vi "MGCC_MdlMgmt_MovetonewMicrogrid.vi"() -> (0 "error out":errorcluster, 1 "error out 2":errorcluster)   [LabVIEW 2016]
uses:
  Global_MdlMgmt.vi
  <vilib>/imath/engines/lvmath2/RunTimeEngine/IndexRead/NIMS M($,R2).vi
  <instcachedir>/0/NIMS M($,R2)_D9380E19261A4ADFB2D364AF6959C6EF.lvgen/NIMS M($,R2)_D9380E19261A4ADFB2D364AF6959C6EF_001.vi
  <vilib>/imath/engines/lvmath2/RunTimeEngine/BuiltInFunctions/max/1 input/NIMS_max(RM).vi
  <instcachedir>/0/NIMS_max(RM)_358AE92FF7FA4D91BF0D9DEC69043403.lvgen/NIMS_max(RM)_358AE92FF7FA4D91BF0D9DEC69043403_000.vi
  <vilib>/imath/engines/lvmath2/RunTimeEngine/BuiltInFunctions/max/1 input/NIMS_max(RV).vi
  <instcachedir>/0/NIMS_max(RV)_237633DB1D604D5BA7001287DF3C7957.lvgen/NIMS_max(RV)_237633DB1D604D5BA7001287DF3C7957_000.vi
  <vilib>/imathl/engines/lvmath/Functions/Error Handling/Create Error.vi
  <vilib>/imath/engines/lvmath2/RunTimeEngine/IndexRead/NIMS M($,S).vi
  <instcachedir>/0/NIMS M($,S)_3E5749BBB62E49528D4765A77F1F6D98.lvgen/NIMS M($,S)_3E5749BBB62E49528D4765A77F1F6D98_000.vi
  <vilib>/imath/engines/lvmath2/RunTimeEngine/BuiltInFunctions/length/NIMS_length(GV).vi
  <instcachedir>/0/NIMS_length(GV)_08A3D13377FD4E4B96F5795FBF3698FA.lvgen/NIMS_length(GV)_08A3D13377FD4E4B96F5795FBF3698FA_000.vi
  <instcachedir>/0/NIMS_length(GV)_08A3D13377FD4E4B96F5795FBF3698FA.lvgen/NIMS_length(GV)_08A3D13377FD4E4B96F5795FBF3698FA_002.vi
  <vilib>/imath/engines/lvmath2/RunTimeEngine/BuiltInFunctions/zeros/NIMS_M=zeros(I32,I32).vi
  <vilib>/imath/engines/lvmath2/RunTimeEngine/ErrorHandling/NIMS_Create Error From Enums.vi
  <vilib>/imath/engines/lvmath2/RunTimeEngine/IndexReplace/NIMS M(S,$)=V.vi
  <instcachedir>/0/NIMS M(S,$)=V_BCCFA522A894489B8FA760383D74A164.lvgen/NIMS M(S,$)=V_BCCFA522A894489B8FA760383D74A164_002.vi
  <vilib>/imath/engines/lvmath2/RunTimeEngine/BuiltInFunctions/zeros/NIMS_V=zeros(I32,I32).vi
  <vilib>/imath/engines/lvmath2/RunTimeEngine/RangeToken/NIMS_Range_R3 - Integer.vi
  <instcachedir>/0/NIMS_Range_R3 - Integer_A435E2FF893B4C718FD5055FE39FE2F6.lvgen/NIMS_Range_R3 - Integer_A435E2FF893B4C718FD5055FE39FE2F6_000.vi
  <vilib>/imath/engines/lvmath2/RunTimeEngine/CommandStatement/MC_CommandStatement_break.vi
  <vilib>/imath/engines/lvmath2/RunTimeEngine/IndexRead/NIMS M(S,R2).vi
  <instcachedir>/0/NIMS M(S,R2)_45730E4D0DB74D118F715F4F99DCE4D7.lvgen/NIMS M(S,R2)_45730E4D0DB74D118F715F4F99DCE4D7_000.vi
  <vilib>/imath/engines/lvmath2/RunTimeEngine/BuiltInFunctions/is_membermx/NIMS_is_membermx(GM,GM).vi
  <instcachedir>/0/NIMS_is_membermx(GM,GM)_DE25F6F493CE4EA1946032CBAF7A49B3.lvgen/NIMS_is_membermx(GM,GM)_DE25F6F493CE4EA1946032CBAF7A49B3_000.vi
  <vilib>/imath/engines/lvmath2/RunTimeEngine/BuiltInFunctions/sum/NIMS_sum(GM,Sca).vi
  <instcachedir>/0/NIMS_sum(GM,Sca)_79BF37D5D11844228B167097B6AFCFEB.lvgen/NIMS_sum(GM,Sca)_79BF37D5D11844228B167097B6AFCFEB_001.vi
  <vilib>/imath/engines/lvmath2/RunTimeEngine/IndexRead/NIMS M(S,S).vi
  <instcachedir>/0/NIMS M(S,S)_AC51E74150A542F7991B9634C66F3096.lvgen/NIMS M(S,S)_AC51E74150A542F7991B9634C66F3096_000.vi
  <vilib>/imath/engines/lvmath2/RunTimeEngine/IndexReplace/NIMS M(S,S)=S.vi
  <instcachedir>/0/NIMS M(S,S)=S_98E40400474E4398B113AE20298B4F82.lvgen/NIMS M(S,S)=S_98E40400474E4398B113AE20298B4F82_000.vi
  <vilib>/imath/engines/lvmath2/RunTimeEngine/BuiltInFunctions/sum/NIMS_sum(GV).vi
  <instcachedir>/0/NIMS_sum(GV)_67F5EC36BC034E54A6BEC5B0673C00E5.lvgen/NIMS_sum(GV)_67F5EC36BC034E54A6BEC5B0673C00E5_000.vi
  <vilib>/imath/engines/lvmath2/RunTimeEngine/BuiltInFunctions/findnz/NIMS_[1o]_findnz(GRowV).vi
  <instcachedir>/0/NIMS_[1o]_findnz(GRowV)_1AF74843B4874134ADE908C0A4A72F3C.lvgen/NIMS_[1o]_findnz(GRowV)_1AF74843B4874134ADE908C0A4A72F3C_000.vi
  <vilib>/imath/engines/lvmath2/RunTimeEngine/IndexRead/NIMS M($,V).vi
  <instcachedir>/0/NIMS M($,V)_706F2CE2C8E141269FD4C8A402E169C5.lvgen/NIMS M($,V)_706F2CE2C8E141269FD4C8A402E169C5_005.vi
  <vilib>/imath/engines/lvmath2/RunTimeSupport/NIMS_Get Any Vector_w Error - Matrix.vi
  <instcachedir>/0/NIMS_Get Any Vector_w Error - Matrix_2B7BCBEFD1FA4E1C95EFF9244314B21B.lvgen/NIMS_Get Any Vector_w Error - Matrix_2B7BCBEFD1FA4E1C95EFF9244314B21B_001.vi
  <vilib>/imath/engines/lvmath2/RunTimeEngine/BuiltInFunctions/sets_union/NIMS_sets_union(GV2).vi
  <instcachedir>/0/NIMS_sets_union(GV2)_D04DE11E528744D2B40881BC08732835.lvgen/NIMS_sets_union(GV2)_D04DE11E528744D2B40881BC08732835_007.vi
  <vilib>/imath/engines/lvmath2/RunTimeEngine/IndexReplace/NIMS M($,V)=V.vi
  <instcachedir>/0/NIMS M($,V)=V_456DED019FC24BEA8A1C4EECB3220DB5.lvgen/NIMS M($,V)=V_456DED019FC24BEA8A1C4EECB3220DB5_000.vi
  <vilib>/imath/engines/lvmath2/RunTimeEngine/RangeToken/NIMS_Range.vi
  <instcachedir>/0/NIMS_Range_A7C094595B484CA7AF10685B02D808ED.lvgen/NIMS_Range_A7C094595B484CA7AF10685B02D808ED_001.vi
  <vilib>/imath/engines/lvmath2/RunTimeEngine/NodeEndStatement/NIMS_NodeEndStatement_Output.vi
  <instcachedir>/0/NIMS_NodeEndStatement_Output_53EC0D466D134D7ABD903AC30B43404B.lvgen/NIMS_NodeEndStatement_Output_53EC0D466D134D7ABD903AC30B43404B_002.vi
  <instcachedir>/0/NIMS_NodeEndStatement_Output_53EC0D466D134D7ABD903AC30B43404B.lvgen/NIMS_NodeEndStatement_Output_53EC0D466D134D7ABD903AC30B43404B_011.vi
  <vilib>/imath/engines/lvmath2/RunTimeEngine/ErrorHandling/NIMS_Finalize Error.vi
  <vilib>/Utility/error.llb/Error Cluster From Error Code.vi
  <vilib>/ErrorRing/Error Ring.xnode
panel:
  out "subarray":cdb[](array[numeric])
  out "Nodematrix":dbl[][](array[numeric])
  out "island_number":i32
  out "Microgrid Topology Overall":dbl[][](array[numeric])
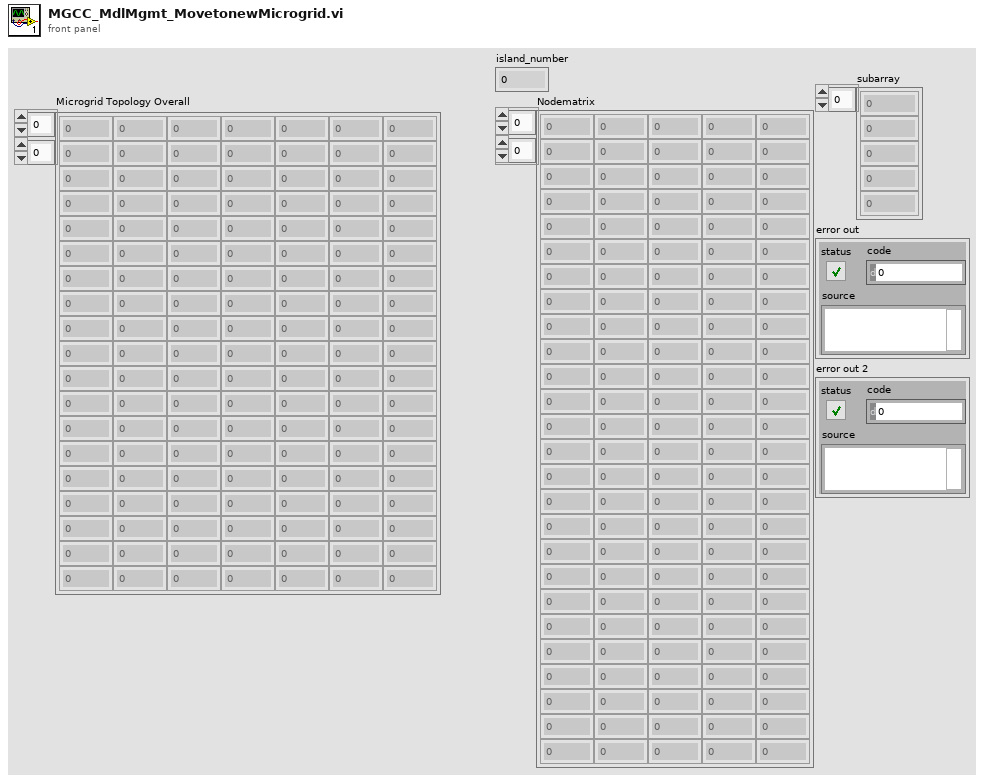
[diagram p1: front panel]
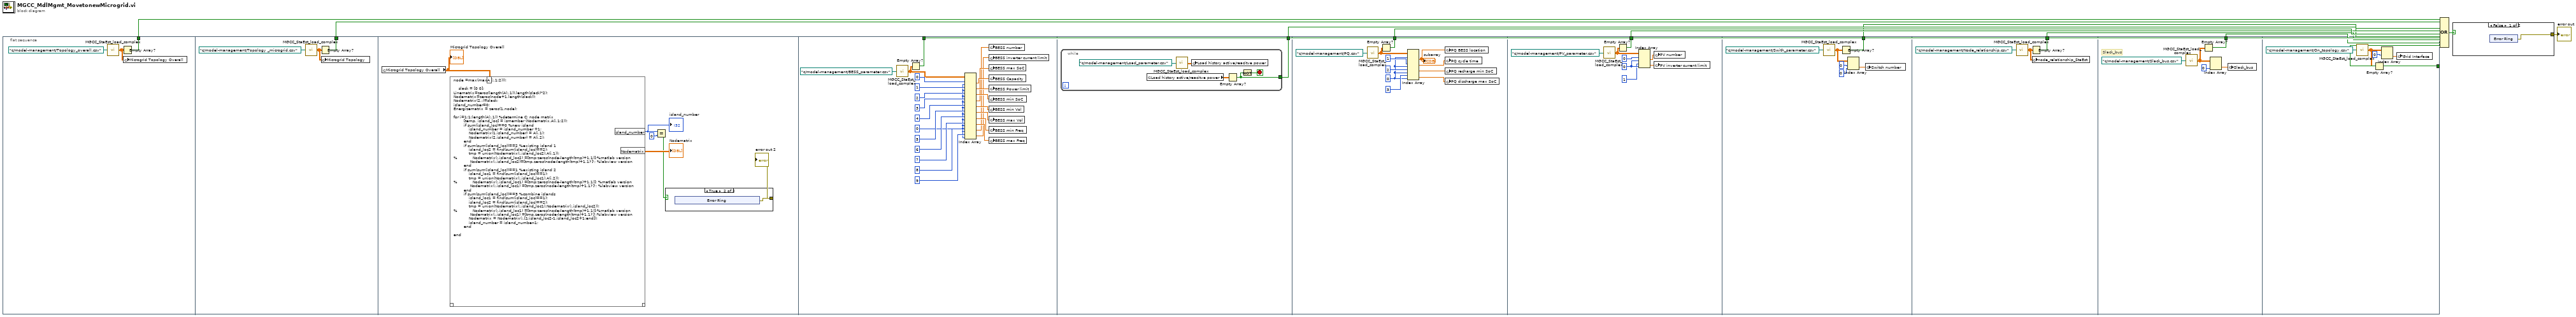
[diagram p0: block diagram]
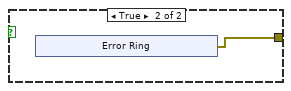
[diagram p2: hidden frame]
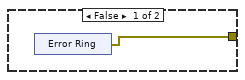
[diagram p3: hidden frame]
diagram:
  n1 = flat-sequence {
    tunnel: [w13] -> w12
    tunnel: [w16] -> w11
    tunnel: [w756] -> w10
    tunnel: [w780] -> w9
    tunnel: [w786] -> w7
    tunnel: [w797] -> w6
    tunnel: [w805] -> w5
    tunnel: [w811] -> w4
    tunnel: [w814] -> w3
    tunnel: [w819] -> w2
    frame #0 {
      n2 = call "MGCC_StaEst_load_complex.vi"("file path (dialog if empty)"=path "c:/model-management/Topology_overall.csv" ("file path (use dialog)")) -> ("Array 13"=w14:cdb[][])
      n3 = Empty Array?(array=w14) -> (empty?=w13:bool)
      n4 = global write "Global_MdlMgmt.vi" "Microgrid Topology Overall"(w14) -> ()
    }
    frame #1 {
      n5 = call "MGCC_StaEst_load_complex.vi"("file path (dialog if empty)"=path "c:/model-management/Topology _microgrid.csv" ("file path (use dialog)")) -> ("Array 13"=w17:cdb[][])
      n6 = Empty Array?(array=w17) -> (empty?=w16:bool)
      n7 = global write "Global_MdlMgmt.vi" "Microgrid Topology"(w17) -> ()
    }
    frame #2 {
      n8 = global read "Global_MdlMgmt.vi" "Microgrid Topology Overall"() -> (w24:dbl[][])
      "Microgrid Topology Overall" <- w24
      n9 = mathscript code="node =max(max(A(:,1:2)));\n\n    slack = [0 0];\nLinematrix=zeros(length(A(:,1)),length(slack)*2);\nNodematrix=zeros(node+1,length(slack));\nNodematrix(2,:)=slack;\nisland_number=0;\nEnergizematrix = zeros(1,node);\n\nfor i=1:1:length(A(:,1)) %determine C: node matrix\n        [temp, island_loc] = ismember (Nodematrix,A(i,1:2));\n        if sum(island_loc)==0 %new island\n            island_number = island_number +1;\n            Nodematrix(1,island_number) = A(i,1);\n            Nodematrix(2,island_number) = A(i,2);\n        end\n        if sum(sum(island_loc))==2 %existing island 1\n            island_loc2 = find(sum(island_loc)==2);\n            tmp = union(Nodematrix(:,island_loc2),A(i,1));\n%            Nodematrix(:,island_loc2) =[tmp;zeros(node-length(tmp)+1,1)];%matlab version\n             Nodematrix(:,island_loc2)=[tmp,zeros(node-length(tmp)+1,1)']'; %labview version\n        end\n        if sum(sum(island_loc))==1 %existing island 2\n            island_loc1 = find(sum(island_loc)==1);\n            tmp = union(Nodematrix(:,island_loc1),A(i,2));\n%            Nodematrix(:,island_loc1) =[tmp;zeros(node-length(tmp)+1,1)]; %matlab version\n             Nodematrix(:,island_loc1) =[tmp,zeros(node-length(tmp)+1,1)']'; %labview version\n        end\n        if sum(sum(island_loc))==3 %combine islands\n            island_loc1 = find(sum(island_loc)==1);\n            island_loc2 = find(sum(island_loc)==2);\n            tmp = union(Nodematrix(:,island_loc1),Nodematrix(:,island_loc2));\n%            Nodematrix(:,island_loc1) =[tmp;zeros(node-length(tmp)+1,1)];%matlab version\n             Nodematrix(:,island_loc1) =[tmp,zeros(node-length(tmp)+1,1)']';%labview version\n            Nodematrix = Nodematrix(:,[1:island_loc2-1,island_loc2+1:end]);\n            island_number = island_number-1;\n        end\n\nend"("A"=w24) -> ("island_number"=w22:i32, "Nodematrix"=→"Nodematrix":dbl[][])  [unwired: 1 in, 1 out]
      "island_number" <- w22
      n10 = Equal?(x=w22, y=0) -> (x = y?=w20:bool)
      n11 = case shown="True" w20 {
        tunnel: [w25 w27] -> w19
        frame False {
          n12 = xnode "Error Ring"() -> ("error out"=w25:errorcluster)
        }
        frame True {
          n13 = xnode "Error Ring"() -> ("error out"=w27:errorcluster)
        }
      }
      "error out 2" <- w19
    }
    frame #3 {
      w768 = 0
      n14 = call "MGCC_StaEst_load_complex.vi"("file path (dialog if empty)"=path "c:/model-management/BESS_parameter.csv" ("file path (use dialog)")) -> ("Array 13"=w757:cdb[][])
      n15 = Empty Array?(array=w757) -> (empty?=w756:bool)
      n16 = Index Array(array=w757, index (row) #1=0 ("disabled index (row)"), index (col) #1=w768, index (row) #2=1 ("disabled index (row)"), index (col) #2=w768, index (row) #3=2 ("disabled index (row)"), index (col) #3=w768, index (row) #4=3 ("disabled index (row)"), index (col) #4=w768, index (row) #5=4 ("disabled index (row)"), index (col) #5=w768, index (row) #6=5 ("disabled index (row)"), index (col) #6=w768, index (row) #7=6 ("disabled index (row)"), index (col) #7=w768, index (row) #8=7 ("index (row)"), index (col) #8=w768, index (row) #9=8 ("index (row)"), index (col) #9=w768, index (row) #10=9 ("index (row)"), index (col) #10=w768) -> (element #1=w767:cdb, element #2=w766:cdb, element #3=w765:cdb, element #4=w764:cdb, element #5=w763:cdb, element #6=w762:cdb, element #7=w761:cdb, element #8=w760:cdb, element #9=w759:cdb, element #10=w758:cdb)
      n17 = global write "Global_MdlMgmt.vi" "BESS number"(w759) -> ()
      n18 = global write "Global_MdlMgmt.vi" "BESS inverter current limit"(w758) -> ()
      n19 = global write "Global_MdlMgmt.vi" "BESS max SoC"(w764) -> ()
      n20 = global write "Global_MdlMgmt.vi" "BESS Capacity"(w767) -> ()
      n21 = global write "Global_MdlMgmt.vi" "BESS Power limit"(w766) -> ()
      n22 = global write "Global_MdlMgmt.vi" "BESS min SoC"(w765) -> ()
      n23 = global write "Global_MdlMgmt.vi" "BESS min Vol"(w763) -> ()
      n24 = global write "Global_MdlMgmt.vi" "BESS max Vol"(w762) -> ()
      n25 = global write "Global_MdlMgmt.vi" "BESS min Freq"(w761) -> ()
      n26 = global write "Global_MdlMgmt.vi" "BESS max Freq"(w760) -> ()
    }
    frame #4 {
      n27 = while {
        tunnel: [w781] -> w780
        stop <- w782 stop-if-true
        n28 = global read "Global_MdlMgmt.vi" "Load history active/reacitve power"() -> (w783:dbl[][])
        n29 = call "MGCC_StaEst_load_complex.vi"("file path (dialog if empty)"=path "c:/model-management/Load_parameter.csv" ("file path (use dialog)")) -> ("Array 13"=w784:cdb[][])
        n30 = global write "Global_MdlMgmt.vi" "Load history active/reacitve power"(w784) -> ()
        n31 = Empty Array?(array=w783) -> (empty?=w781:bool)
        n32 = Not(x=w781) -> (.not. x?=w782:bool)
      }
    }
    frame #5 {
      w788 = 0
      n33 = call "MGCC_StaEst_load_complex.vi"("file path (dialog if empty)"=path "c:/model-management/PQ.csv" ("file path (use dialog)")) -> ("Array 13"=w787:cdb[][])
      n34 = Empty Array?(array=w787) -> (empty?=w786:bool)
      n35 = Index Array(array=w787, index (row) #1=w788, index (row) #2=1 ("disabled index (row)"), index (col) #2=w788, index (row) #3=2 ("disabled index (row)"), index (col) #3=w788, index (row) #4=3 ("disabled index (row)"), index (col) #4=w788) -> (element #1=w792:cdb[], element #2=w791:cdb, element #3=w790:cdb, element #4=w789:cdb)  [unwired: 1 in]
      "subarray" <- w792
      n36 = global write "Global_MdlMgmt.vi" "PQ BESS location"(w792) -> ()
      n37 = global write "Global_MdlMgmt.vi" "PQ cycle time"(w791) -> ()
      n38 = global write "Global_MdlMgmt.vi" "PQ recharge min SoC"(w790) -> ()
      n39 = global write "Global_MdlMgmt.vi" "PQ discharge max SoC"(w789) -> ()
    }
    frame #6 {
      w803 = 0
      n40 = call "MGCC_StaEst_load_complex.vi"("file path (dialog if empty)"=path "c:/model-management/PV_parameter.csv" ("file path (use dialog)")) -> ("Array 13"=w798:cdb[][])
      n41 = Empty Array?(array=w798) -> (empty?=w797:bool)
      n42 = Index Array(array=w798, index (row) #1=0 ("disabled index (row)"), index (col) #1=w803, index (row) #2=1 ("disabled index (row)"), index (col) #2=w803) -> (element #1=w800:cdb, element #2=w799:cdb)
      n43 = global write "Global_MdlMgmt.vi" "PV number"(w800) -> ()
      n44 = global write "Global_MdlMgmt.vi" "PV inverter current limit"(w799) -> ()
    }
    frame #7 {
      n45 = call "MGCC_StaEst_load_complex.vi"("file path (dialog if empty)"=path "c:/model-management/Swith_parameter.csv" ("file path (use dialog)")) -> ("Array 13"=w806:cdb[][])
      n46 = Empty Array?(array=w806) -> (empty?=w805:bool)
      n47 = Index Array(array=w806, index (row)=0, index (col)=0 ("disabled index (col)")) -> (element=w807:cdb)
      n48 = global write "Global_MdlMgmt.vi" "Switch number"(w807) -> ()
    }
    frame #8 {
      n49 = call "MGCC_StaEst_load_complex.vi"("file path (dialog if empty)"=path "c:/model-management/Node_relationship.csv" ("file path (use dialog)")) -> ("Array 13"=w812:cdb[][])
      n50 = Empty Array?(array=w812) -> (empty?=w811:bool)
      n51 = global write "Global_MdlMgmt.vi" "node_relationship_StaEst"(w812) -> ()
    }
    frame #9 {
      # "Slack_bus"
      n52 = call "MGCC_StaEst_load_complex.vi"("file path (dialog if empty)"=path "c:/model-management/Slack_bus.csv" ("file path (use dialog)")) -> ("Array 13"=w815:cdb[][])
      n53 = Empty Array?(array=w815) -> (empty?=w814:bool)
      n54 = Index Array(array=w815, index (col)=0 ("disabled index (col)")) -> (element=w816:cdb[])  [unwired: 1 in]
      n55 = global write "Global_MdlMgmt.vi" "Slack_bus"(w816) -> ()
    }
    frame #10 {
      n56 = call "MGCC_StaEst_load_complex.vi"("file path (dialog if empty)"=path "c:/model-management/On_topology.csv" ("file path (use dialog)")) -> ("Array 13"=w820:cdb[][])
      n57 = Empty Array?(array=w820) -> (empty?=w819:bool)
      n58 = Index Array(array=w820, index (row)=0) -> (element=w822:cdb[])  [unwired: 1 in]
      n59 = global write "Global_MdlMgmt.vi" "Grid Interface"(w822) -> ()
    }
  }
  n60 = Compound Arithmetic op=OR(w12, w11, w10, w9, w6, w7, w5, w4, w3, w2) -> (w8:bool)
  n61 = case shown="False" w8 {
    tunnel: [w824 w826] -> w1
    frame False {
      n62 = xnode "Error Ring"() -> ("error out"=w824:errorcluster)
    }
    frame True {
      n63 = xnode "Error Ring"() -> ("error out"=w826:errorcluster)
    }
  }
  "error out" <- w1
